vi "Format CSV.vi"(8 "error in (no error)":errorcluster, 9 "delimiter":string=",", 10 "CSV File Input":path, 11 "Original CSV Format":enum16{"Format A", "Format B"}(ring)) -> (0 "error out":errorcluster, 1 "Parcel Length":i32[](array[numeric]), 2 "All Terminal Data":T1(array[cluster]))   [LabVIEW 2017] (continued)
, "42:48.2", "42:48.2", "42:48.3", "42:48.3", "42:48.3", "42:48.4", "42:48.4", "42:48.4", "42:48.5", "42:48.5", "42:48.5", "42:48.6", "42:48.6", "42:48.6", "42:48.7", "42:48.7", "42:48.7", "42:48.8", "42:48.8", "42:48.8", "42:48.9", "42:48.9", "42:48.9", "42:49.0", "42:49.0", "42:49.0", "42:49.1", "42:49.1", "42:49.1", "42:49.2", "42:49.2", "42:49.2", "42:49.3", "42:49.3", "42:49.3", "42:49.4", "42:49.4", "42:49.4", "42:49.5", "42:49.5", "42:49.5", "42:49.6", "42:49.6", "42:49.6", "42:49.7", "42:49.7", "42:49.7", "42:49.8", "42:49.8", "42:49.8", "42:49.9", "42:49.9", "42:49.9", "42:50.0", "42:50.0", "42:50.0", "42:50.1", "42:50.1", "42:50.1", "42:50.2", "42:50.2", "42:50.2", "42:50.3", "42:50.3", "42:50.3", "42:50.4", "42:50.4", "42:50.4", "42:50.5", "42:50.5", "42:50.5", "42:50.6", "42:50.6", "42:50.6", "42:50.7", "42:50.7", "42:50.7", "42:50.8", "42:50.8", "42:50.8", "42:50.9", "42:50.9", "42:50.9", "42:51.0", "42:51.0", "42:51.0", "42:51.1", "42:51.1", "42:51.1", "42:51.2", "42:51.2", "42:51.2", "42:51.3", "42:51.3", "42:51.3", "42:51.4", "42:51.4", "42:51.4", "42:51.5", "42:51.5", "42:51.5", "42:51.6", "42:51.6", "42:51.6", "42:51.7", "42:51.7", "42:51.7", "42:51.8", "42:51.8", "42:51.8", "42:51.9", "42:51.9", "42:51.9", "42:52.0", "42:52.0", "42:52.0", "42:52.1", "42:52.1", "42:52.1", "42:52.2", "42:52.2", "42:52.2", "42:52.3", "42:52.3", "42:52.3", "42:52.4", "42:52.4", "42:52.4", "42:52.5", "42:52.5", "42:52.5", "42:52.6", "42:52.6", "42:52.6", "42:52.7", "42:52.7", "42:52.7", "42:52.8", "42:52.8", "42:52.8", "42:52.9", "42:52.9", "42:52.9", "42:53.0", "42:53.0", "42:53.0", "42:53.1", "42:53.1", "42:53.1", "42:53.2", "42:53.2", "42:53.2", "42:53.3", "42:53.3", "42:53.3", "42:53.4", "42:53.4", "42:53.4", "42:53.5", "42:53.5", "42:53.5", "42:53.6", "42:53.6", "42:53.6", "42:53.7", "42:53.7", "42:53.7", "42:53.8", "42:53.8", "42:53.8", "42:53.9", "42:53.9", "42:53.9", "42:54.0", "42:54.0", "42:54.0", "42:54.1", "42:54.1", "42:54.1", "42:54.2", "42:54.2", "42:54.2", "42:54.3", "42:54.3", "42:54.3", "42:54.4", "42:54.4", "42:54.4", "42:54.5", "42:54.5", "42:54.5", "42:54.6", "42:54.6", "42:54.6", "42:54.7", "42:54.7", "42:54.7", "42:54.8", "42:54.8", "42:54.8", "42:54.9", "42:54.9", "42:54.9", "42:55.0", "42:55.0", "42:55.0", "42:55.1", "42:55.1", "42:55.1", "42:55.2", "42:55.2", "42:55.2", "42:55.3", "42:55.3", "42:55.3", "42:55.4", "42:55.4", "42:55.4", "42:55.5", "42:55.5", "42:55.5", "42:55.6", "42:55.6", "42:55.6", "42:55.7", "42:55.7", "42:55.7", "42:55.8", "42:55.8", "42:55.8", "42:55.9", "42:55.9", "42:55.9", "42:56.0", "42:56.0", "42:56.0", "42:56.1", "42:56.1", "42:56.1", "42:56.2", "42:56.2", "42:56.2", "42:56.3", "42:56.3", "42:56.3", "42:56.4", "42:56.4", "42:56.4", "42:56.5", "42:56.5", "42:56.5", "42:56.6", "42:56.6", "42:56.6", "42:56.7", "42:56.7", "42:56.7", "42:56.8", "42:56.8", "42:56.8", "42:56.9", "42:56.9", "42:56.9", "42:57.0", "42:57.0", "42:57.0", "42:57.1", "42:57.1", "42:57.1", "42:57.2", "42:57.2", "42:57.2", "42:57.3", "42:57.3", "42:57.3", "42:57.4", "42:57.4", "42:57.4", "42:57.5", "42:57.5", "42:57.5", "42:57.6", "42:57.6", "42:57.6", "42:57.7", "42:57.7", "42:57.7", "42:57.8", "42:57.8", "42:57.8", "42:57.9", "42:57.9", "42:57.9", "42:58.0", "42:58.0", "42:58.0", "42:58.1", "42:58.1", "42:58.1", "42:58.2", "42:58.2", "42:58.2", "42:58.3", "42:58.3", "42:58.3", "42:58.4", "42:58.4", "42:58.4", "42:58.5", "42:58.5", "42:58.5", "42:58.6", "42:58.6", "42:58.6", "42:58.7", "42:58.7", "42:58.7", "42:58.8", "42:58.8", "42:58.8", "42:58.9", "42:58.9", "42:58.9", "42:59.0", "42:59.0", "42:59.0", "42:59.1", "42:59.1", "42:59.1", "42:59.2", "42:59.2", "42:59.2", "42:59.3", "42:59.3", "42:59.3", "42:59.4", "42:59.4", "42:59.4", "42:59.5", "42:59.5", "42:59.5", "42:59.6", "42:59.6", "42:59.6", "42:59.7", "42:59.7", "42:59.7", "42:59.8", "42:59.8", "42:59.8", "42:59.9", "42:59.9", "42:59.9", "43:00.0", "43:00.0", "43:00.0", "43:00.1", "43:00.1", "43:00.1", "43:00.2", "43:00.2", "43:00.2", "43:00.3", "43:00.3", "43:00.3", "43:00.4", "43:00.4", "43:00.4", "43:00.5", "43:00.5", "43:00.5", "43:00.6", "43:00.6", "43:00.6", "43:00.7", "43:00.7", "43:00.7", "43:00.8", "43:00.8", "43:00.8", "43:00.9", "43:00.9", "43:00.9", "43:01.0", "43:01.0", "43:01.0", "43:01.1", "43:01.1", "43:01.1", "43:01.2", "43:01.2", "43:01.2", "43:01.3", "43:01.3", "43:01.3", "43:01.4", "43:01.4", "43:01.4", "43:01.5", "43:01.5", "43:01.5", "43:01.6", "43:01.6", "43:01.6", "43:01.7", "43:01.7", "43:01.7", "43:01.8", "43:01.8", "43:01.8", "43:01.9", "43:01.9", "43:01.9", "43:02.0", "43:02.0", "43:02.0", "43:02.1", "43:02.1", "43:02.1", "43:02.2", "43:02.2", "43:02.2", "43:02.3", "43:02.3", "43:02.3", "43:02.4", "43:02.4", "43:02.4", "43:02.5", "43:02.5", "43:02.5", "43:02.6", "43:02.6", "43:02.6", "43:02.7", "43:02.7", "43:02.7", "43:02.8", "43:02.8", "43:02.8", "43:02.9", "43:02.9", "43:02.9", "43:03.0", "43:03.0", "43:03.0", "43:03.1", "43:03.1", "43:03.1", "43:03.2", "43:03.2", "43:03.2", "43:03.3", "43:03.3", "43:03.3", "43:03.4", "43:03.4", "43:03.4", "43:03.5", "43:03.5", "43:03.5", "43:03.6", "43:03.6", "43:03.6", "43:03.7", "43:03.7", "43:03.7", "43:03.8", "43:03.8", "43:03.8", "43:03.9", "43:03.9", "43:03.9", "43:04.0", "43:04.0", "43:04.0", "43:04.1", "43:04.1", "43:04.1", "43:04.2", "43:04.2", "43:04.2", "43:04.3", "43:04.3", "43:04.3", "43:04.4", "43:04.4", "43:04.4", "43:04.5", "43:04.5", "43:04.5", "43:04.6", "43:04.6", "43:04.6", "43:04.7", "43:04.7", "43:04.7", "43:04.8", "43:04.8", "43:04.8", "43:04.9", "43:04.9", "43:04.9", "43:05.0", "43:05.0", "43:05.0", "43:05.1", "43:05.1", "43:05.1", "43:05.2", "43:05.2", "43:05.2", "43:05.3", "43:05.3", "43:05.3", "43:05.4", "43:05.4", "43:05.4", "43:05.5", "43:05.5", "43:05.5", "43:05.6", "43:05.6", "43:05.6", "43:05.7", "43:05.7", "43:05.7", "43:05.8", "43:05.8", "43:05.8", "43:05.9", "43:05.9", "43:05.9", "43:06.0", "43:06.0", "43:06.0", "43:06.1", "43:06.1", "43:06.1", "43:06.2", "43:06.2", "43:06.2", "43:06.3", "43:06.3", "43:06.3", "43:06.4", "43:06.4", "43:06.4", "43:06.5", "43:06.5", "43:06.5", "43:06.6", "43:06.6", "43:06.6", "43:06.7", "43:06.7", "43:06.7", "43:06.8", "43:06.8", "43:06.8", "43:06.9", "43:06.9", "43:06.9", "43:07.0", "43:07.0", "43:07.0", "43:07.1", "43:07.1", "43:07.1", "43:07.2", "43:07.2", "43:07.2", "43:07.3", "43:07.3", "43:07.3", "43:07.4", "43:07.4", "43:07.4", "43:07.5", "43:07.5", "43:07.5", "43:07.6", "43:07.6", "43:07.6", "43:07.7", "43:07.7", "43:07.7", "43:07.8", "43:07.8", "43:07.8", "43:07.9", "43:07.9", "43:07.9", "43:08.0", "43:08.0", "43:08.0", "43:08.1", "43:08.1", "43:08.1", "43:08.2", "43:08.2", "43:08.2", "43:08.3", "43:08.3", "43:08.3", "43:08.4", "43:08.4", "43:08.4", "43:08.5", "43:08.5", "43:08.5", "43:08.6", "43:08.6", "43:08.6", "43:08.7", "43:08.7", "43:08.7", "43:08.8", "43:08.8", "43:08.8", "43:08.9", "43:08.9", "43:08.9", "43:09.0", "43:09.0", "43:09.0", "43:09.1", "43:09.1", "43:09.1", "43:09.2", "43:09.2", "43:09.2", "43:09.3", "43:09.3", "43:09.3", "43:09.4", "43:09.4", "43:09.4", "43:09.5", "43:09.5", "43:09.5", "43:09.6", "43:09.6", "43:09.6", "43:09.7", "43:09.7", "43:09.7", "43:09.8", "43:09.8", "43:09.8", "43:09.9", "43:09.9", "43:09.9", "43:10.0", "43:10.0", "43:10.0", "43:10.1", "43:10.1", "43:10.1", "43:10.2", "43:10.2", "43:10.2", "43:10.3", "43:10.3", "43:10.3", "43:10.4", "43:10.4", "43:10.4", "43:10.5", "43:10.5", "43:10.5", "43:10.6", "43:10.6", "43:10.6", "43:10.7", "43:10.7", "43:10.7", "43:10.8", "43:10.8", "43:10.8", "43:10.9", "43:10.9", "43:10.9", "43:11.0", "43:11.0", "43:11.0", "43:11.1", "43:11.1", "43:11.1", "43:11.2", "43:11.2", "43:11.2", "43:11.3", "43:11.3", "43:11.3", "43:11.4", "43:11.4", "43:11.4", "43:11.5", "43:11.5", "43:11.5", "43:11.6", "43:11.6", "43:11.6", "43:11.7", "43:11.7", "43:11.7", "43:11.8", "43:11.8", "43:11.8", "43:11.9", "43:11.9", "43:11.9", "43:12.0", "43:12.0", "43:12.0", "43:12.1", "43:12.1", "43:12.1", "43:12.2", "43:12.2", "43:12.2", "43:12.3", "43:12.3", "43:12.3", "43:12.4", "43:12.4", "43:12.4", "43:12.5", "43:12.5", "43:12.5", "43:12.6", "43:12.6", "43:12.6", "43:12.7", "43:12.7", "43:12.7", "43:12.8", "43:12.8", "43:12.8", "43:12.9", "43:12.9", "43:12.9", "43:13.0", "43:13.0", "43:13.0", "43:13.1", "43:13.1", "43:13.1", "43:13.2", "43:13.2", "43:13.2", "43:13.3", "43:13.3", "43:13.3", "43:13.4", "43:13.4", "43:13.4", "43:13.5", "43:13.5", "43:13.5", "43:13.6", "43:13.6", "43:13.6", "43:13.7", "43:13.7", "43:13.7", "43:13.8", "43:13.8", "43:13.8", "43:13.9", "43:13.9", "43:13.9", "43:14.0", "43:14.0", "43:14.0", "43:14.1", "43:14.1", "43:14.1", "43:14.2", "43:14.2", "43:14.2", "43:14.3", "43:14.3", "43:14.3", "43:14.4", "43:14.4", "43:14.4", "43:14.5", "43:14.5", "43:14.5", "43:14.6", "43:14.6", "43:14.6", "43:14.7", "43:14.7", "43:14.7", "43:14.8", "43:14.8", "43:14.8", "43:14.9", "43:14.9", "43:14.9", "43:15.0", "43:15.0", "43:15.0", "43:15.1", "43:15.1", "43:15.1", "43:15.2", "43:15.2", "43:15.2", "43:15.3", "43:15.3", "43:15.3", "43:15.4", "43:15.4", "43:15.4", "43:15.5", "43:15.5", "43:15.5", "43:15.6", "43:15.6", "43:15.6", "43:15.7", "43:15.7", "43:15.7", "43:15.8", "43:15.8", "43:15.8", "43:15.9", "43:15.9", "43:15.9", "43:16.0", "43:16.0", "43:16.0", "43:16.1", "43:16.1", "43:16.1", "43:16.2", "43:16.2", "43:16.2", "43:16.3", "43:16.3", "43:16.3", "43:16.4", "43:16.4", "43:16.4", "43:16.5", "43:16.5", "43:16.5", "43:16.6", "43:16.6", "43:16.6", "43:16.7", "43:16.7", "43:16.7", "43:16.8", "43:16.8", "43:16.8", "43:16.9", "43:16.9", "43:16.9", "43:17.0", "43:17.0", "43:17.0", "43:17.1", "43:17.1", "43:17.1", "43:17.2", "43:17.2", "43:17.2", "43:17.3", "43:17.3", "43:17.3", "43:17.4", "43:17.4", "43:17.4", "43:17.5", "43:17.5", "43:17.5", "43:17.6", "43:17.6", "43:17.6", "43:17.7", "43:17.7", "43:17.7", "43:17.8", "43:17.8", "43:17.8", "43:17.9", "43:17.9", "43:17.9", "43:18.0", "43:18.0", "43:18.0", "43:18.1", "43:18.1", "43:18.1", "43:18.2", "43:18.2", "43:18.2", "43:18.3", "43:18.3", "43:18.3", "43:18.4", "43:18.4", "43:18.4", "43:18.5", "43:18.5", "43:18.5", "43:18.6", "43:18.6", "43:18.6", "43:18.7", "43:18.7", "43:18.7", "43:18.8", "43:18.8", "43:18.8", "43:18.9", "43:18.9", "43:18.9", "43:19.0", "43:19.0", "43:19.0", "43:19.1", "43:19.1", "43:19.1", "43:19.2", "43:19.2", "43:19.2", "43:19.3", "43:19.3", "43:19.3", "43:19.4", "43:19.4", "43:19.4", "43:19.5", "43:19.5", "43:19.5", "43:19.6", "43:19.6", "43:19.6", "43:19.7", "43:19.7", "43:19.7", "43:19.8", "43:19.8", "43:19.8", "43:19.9", "43:19.9", "43:19.9", "43:20.0", "43:20.0", "43:20.0", "43:20.1", "43:20.1", "43:20.1", "43:20.2", "43:20.2", "43:20.2", "43:20.3", "43:20.3", "43:20.3", "43:20.4", "43:20.4", "43:20.4", "43:20.5", "43:20.5", "43:20.5", "43:20.6", "43:20.6", "43:20.6", "43:20.7", "43:20.7", "43:20.7", "43:20.8", "43:20.8", "43:20.8", "43:20.9", "43:20.9", "43:20.9", "43:21.0", "43:21.0", "43:21.0", "43:21.1", "43:21.1", "43:21.1", "43:21.2", "43:21.2", "43:21.2", "43:21.3", "43:21.3", "43:21.3", "43:21.4", "43:21.4", "43:21.4", "43:21.5", "43:21.5", "43:21.5", "43:21.6", "43:21.6", "43:21.6", "43:21.7", "43:21.7", "43:21.7", "43:21.8", "43:21.8", "43:21.8", "43:21.9", "43:21.9", "43:21.9", "43:22.0", "43:22.0", "43:22.0", "43:22.1", "43:22.1", "43:22.1", "43:22.2", "43:22.2", "43:22.2", "43:22.3", "43:22.3", "43:22.3", "43:22.4", "43:22.4", "43:22.4", "43:22.5", "43:22.5", "43:22.5", "43:22.6", "43:22.6", "43:22.6", "43:22.7", "43:22.7", "43:22.7", "43:22.8", "43:22.8", "43:22.8", "43:22.9", "43:22.9", "43:22.9", "43:23.0", "43:23.0", "43:23.0", "43:23.1", "43:23.1", "43:23.1", "43:23.2", "43:23.2", "43:23.2", "43:23.3", "43:23.3", "43:23.3", "43:23.4", "43:23.4", "43:23.4", "43:23.5", "43:23.5", "43:23.5", "43:23.6", "43:23.6", "43:23.6", "43:23.7", "43:23.7", "43:23.7", "43:23.8", "43:23.8", "43:23.8", "43:23.9", "43:23.9", "43:23.9", "43:24.0", "43:24.0", "43:24.0", "43:24.1", "43:24.1", "43:24.1", "43:24.2", "43:24.2", "43:24.2", "43:24.3", "43:24.3", "43:24.3", "43:24.4", "43:24.4", "43:24.4", "43:24.5", "43:24.5", "43:24.5", "43:24.6", "43:24.6", "43:24.6", "43:24.7", "43:24.7", "43:24.7", "43:24.8", "43:24.8", "43:24.8", "43:24.9", "43:24.9", "43:24.9", "43:25.0", "43:25.0", "43:25.0", "43:25.1", "43:25.1", "43:25.1", "43:25.2", "43:25.2", "43:25.2", "43:25.3", "43:25.3", "43:25.3", "43:25.4", "43:25.4", "43:25.4", "43:25.5", "43:25.5", "43:25.5", "43:25.6", "43:25.6", "43:25.6", "43:25.7", "43:25.7", "43:25.7", "43:25.8", "43:25.8", "43:25.8", "43:25.9", "43:25.9", "43:25.9", "43:26.0", "43:26.0", "43:26.0", "43:26.1", "43:26.1", "43:26.1", "43:26.2", "43:26.2", "43:26.2", "43:26.3", "43:26.3", "43:26.3", "43:26.4", "43:26.4", "43:26.4", "43:26.5", "43:26.5", "43:26.5", "43:26.6", "43:26.6", "43:26.6", "43:26.7", "43:26.7", "43:26.7", "43:26.8", "43:26.8", "43:26.8", "43:26.9", "43:26.9", "43:26.9", "43:27.0", "43:27.0", "43:27.0", "43:27.1", "43:27.1", "43:27.1", "43:27.2", "43:27.2", "43:27.2", "43:27.3", "43:27.3", "43:27.3", "43:27.4", "43:27.4", "43:27.4", "43:27.5", "43:27.5", "43:27.5", "43:27.6", "43:27.6", "43:27.6", "43:27.7", "43:27.7", "43:27.7", "43:27.8", "43:27.8", "43:27.8", "43:27.9", "43:27.9", "43:27.9", "43:28.0", "43:28.0", "43:28.0", "43:28.1", "43:28.1", "43:28.1", "43:28.2", "43:28.2", "43:28.2", "43:28.3", "43:28.3", "43:28.3", "43:28.4", "43:28.4", "43:28.4", "43:28.5", "43:28.5", "43:28.5", "43:28.6", "43:28.6", "43:28.6", "43:28.7", "43:28.7", "43:28.7", "43:28.8", "43:28.8", "43:28.8", "43:28.9", "43:28.9", "43:28.9", "43:29.0", "43:29.0", "43:29.0", "43:29.1", "43:29.1", "43:29.1", "43:29.2", "43:29.2", "43:29.2", "43:29.3", "43:29.3", "43:29.3", "43:29.4", "43:29.4", "43:29.4", "43:29.5", "43:29.5", "43:29.5", "43:29.6", "43:29.6", "43:29.6", "43:29.7", "43:29.7", "43:29.7", "43:29.8", "43:29.8", "43:29.8", "43:29.9", "43:29.9", "43:29.9", "43:30.0", "43:30.0", "43:30.0", "43:30.1", "43:30.1", "43:30.1", "43:30.2", "43:30.2", "43:30.2", "43:30.3", "43:30.3", "43:30.3", "43:30.4", "43:30.4", "43:30.4", "43:30.5", "43:30.5", "43:30.5", "43:30.6", "43:30.6", "43:30.6", "43:30.7", "43:30.7", "43:30.7", "43:30.8", "43:30.8", "43:30.8", "43:30.9", "43:30.9", "43:30.9", "43:31.0", "43:31.0", "43:31.0", "43:31.1", "43:31.1", "43:31.1", "43:31.2", "43:31.2", "43:31.2", "43:31.3", "43:31.3", "43:31.3", "43:31.4", "43:31.4", "43:31.4", "43:31.5", "43:31.5", "43:31.5", "43:31.6", "43:31.6", "43:31.6", "43:31.7", "43:31.7", "43:31.7", "43:31.8", "43:31.8", "43:31.8", "43:31.9", "43:31.9", "43:31.9", "43:32.0", "43:32.0", "43:32.0", "43:32.1", "43:32.1", "43:32.1", "43:32.2", "43:32.2", "43:32.2", "43:32.3", "43:32.3", "43:32.3", "43:32.4", "43:32.4", "43:32.4", "43:32.5", "43:32.5", "43:32.5", "43:32.6", "43:32.6", "43:32.6", "43:32.7", "43:32.7", "43:32.7", "43:32.8", "43:32.8", "43:32.8", "43:32.9", "43:32.9", "43:32.9", "43:33.0", "43:33.0", "43:33.0", "43:33.1", "43:33.1", "43:33.1", "43:33.2", "43:33.2", "43:33.2", "43:33.3", "43:33.3", "43:33.3", "43:33.4", "43:33.4", "43:33.4", "43:33.5", "43:33.5", "43:33.5", "43:33.6", "43:33.6", "43:33.6", "43:33.7", "43:33.7", "43:33.7", "43:33.8", "43:33.8", "43:33.8", "43:33.9", "43:33.9", "43:33.9", "43:34.0", "43:34.0", "43:34.0", "43:34.1", "43:34.1", "43:34.1", "43:34.2", "43:34.2", "43:34.2", "43:34.3", "43:34.3", "43:34.3", "43:34.4", "43:34.4", "43:34.4", "43:34.5", "43:34.5", "43:34.5", "43:34.6", "43:34.6", "43:34.6", "43:34.7", "43:34.7", "43:34.7", "43:34.8", "43:34.8", "43:34.8", "43:34.9", "43:34.9", "43:34.9", "43:35.0", "43:35.0", "43:35.0", "43:35.1", "43:35.1", "43:35.1", "43:35.2", "43:35.2", "43:35.2", "43:35.3", "43:35.3", "43:35.3", "43:35.4", "43:35.4", "43:35.4", "43:35.5", "43:35.5", "43:35.5", "43:35.6", "43:35.6", "43:35.6", "43:35.7", "43:35.7", "43:35.7", "43:35.8", "43:35.8", "43:35.8", "43:35.9", "43:35.9", "43:35.9", "43:36.0", "43:36.0", "43:36.0", "43:36.1", "43:36.1", "43:36.1", "43:36.2", "43:36.2", "43:36.2", "43:36.3", "43:36.3", "43:36.3", "43:36.4", "43:36.4", "43:36.4", "43:36.5", "43:36.5", "43:36.5", "43:36.6", "43:36.6", "43:36.6", "43:36.7", "43:36.7", "43:36.7", "43:36.8", "43:36.8", "43:36.8", "43:36.9", "43:36.9", "43:36.9", "43:37.0", "43:37.0", "43:37.0", "43:37.1", "43:37.1", "43:37.1", "43:37.2", "43:37.2", "43:37.2", "43:37.3", "43:37.3", "43:37.3", "43:37.4", "43:37.4", "43:37.4", "43:37.5", "43:37.5", "43:37.5", "43:37.6", "43:37.6", "43:37.6", "43:37.7", "43:37.7", "43:37.7", "43:37.8", "43:37.8", "43:37.8", "43:37.9", "43:37.9", "43:37.9", "43:38.0", "43:38.0", "43:38.0", "43:38.1", "43:38.1", "43:38.1", "43:38.2", "43:38.2", "43:38.2", "43:38.3", "43:38.3", "43:38.3", "43:38.4", "43:38.4", "43:38.4", "43:38.5", "43:38.5", "43:38.5", "43:38.6", "43:38.6", "43:38.6", "43:38.7", "43:38.7", "43:38.7", "43:38.8", "43:38.8", "43:38.8", "43:38.9", "43:38.9", "43:38.9", "43:39.0", "43:39.0", "43:39.0", "43:39.1", "43:39.1", "43:39.1", "43:39.2", "43:39.2", "43:39.2", "43:39.3", "43:39.3", "43:39.3", "43:39.4", "43:39.4", "43:39.4", "43:39.5", "43:39.5", "43:39.5", "43:39.6", "43:39.6", "43:39.6", "43:39.7", "43:39.7", "43:39.7", "43:39.8", "43:39.8", "43:39.8", "43:39.9", "43:39.9", "43:39.9", "43:40.0", "43:40.0", "43:40.0", "43:40.1", "43:40.1", "43:40.1", "43:40.2", "43:40.2", "43:40.2", "43:40.3", "43:40.3", "43:40.3", "43:40.4", "43:40.4", "43:40.4", "43:40.5", "43:40.5", "43:40.5", "43:40.6", "43:40.6", "43:40.6", "43:40.7", "43:40.7", "43:40.7", "43:40.8", "43:40.8", "43:40.8", "43:40.9", "43:40.9", "43:40.9", "43:41.0", "43:41.0", "43:41.0", "43:41.1", "43:41.1", "43:41.1", "43:41.2", "43:41.2", "43:41.2", "43:41.3", "43:41.3", "43:41.3", "43:41.4", "43:41.4", "43:41.4", "43:41.5", "43:41.5", "43:41.5", "43:41.6", "43:41.6", "43:41.6", "43:41.7", "43:41.7", "43:41.7", "43:41.8", "43:41.8", "43:41.8", "43:41.9", "43:41.9", "43:41.9", "43:42.0", "43:42.0", "43:42.0", "43:42.1", "43:42.1", "43:42.1", "43:42.2", "43:42.2", "43:42.2", "43:42.3", "43:42.3", "43:42.3", "43:42.4", "43:42.4", "43:42.4", "43:42.5", "43:42.5", "43:42.5", "43:42.6", "43:42.6", "43:42.6", "43:42.7", "43:42.7", "43:42.7", "43:42.8", "43:42.8", "43:42.8", "43:42.9", "43:42.9", "43:42.9", "43:43.0", "43:43.0", "43:43.0", "43:43.1", "43:43.1", "43:43.1", "43:43.2", "43:43.2", "43:43.2", "43:43.3", "43:43.3", "43:43.3", "43:43.4", "43:43.4", "43:43.4", "43:43.5", "43:43.5", "43:43.5", "43:43.6", "43:43.6", "43:43.6", "43:43.7", "43:43.7", "43:43.7", "43:43.8", "43:43.8", "43:43.8", "43:43.9", "43:43.9", "43:43.9", "43:44.0", "43:44.0", "43:44.0", "43:44.1", "43:44.1", "43:44.1", "43:44.2", "43:44.2", "43:44.2", "43:44.3", "43:44.3", "43:44.3", "43:44.4", "43:44.4", "43:44.4", "43:44.5", "43:44.5", "43:44.5", "43:44.6", "43:44.6", "43:44.6", "43:44.7", "43:44.7", "43:44.7", "43:44.8", "43:44.8", "43:44.8", "43:44.9", "43:44.9", "43:44.9", "43:45.0", "43:45.0", "43:45.0", "43:45.1", "43:45.1", "43:45.1", "43:45.2", "43:45.2", "43:45.2", "43:45.3", "43:45.3", "43:45.3", "43:45.4", "43:45.4", "43:45.4", "43:45.5", "43:45.5", "43:45.5", "43:45.6", "43:45.6", "43:45.6", "43:45.7", "43:45.7", "43:45.7", "43:45.8", "43:45.8", "43:45.8", "43:45.9", "43:45.9", "43:45.9", "43:46.0", "43:46.0", "43:46.0", "43:46.1", "43:46.1", "43:46.1", "43:46.2", "43:46.2", "43:46.2", "43:46.3", "43:46.3", "43:46.3", "43:46.4", "43:46.4", "43:46.4", "43:46.5", "43:46.5", "43:46.5", "43:46.6", "43:46.6", "43:46.6", "43:46.7", "43:46.7", "43:46.7", "43:46.8", "43:46.8", "43:46.8", "43:46.9", "43:46.9", "43:46.9", "43:47.0", "43:47.0", "43:47.0", "43:47.1", "43:47.1", "43:47.1", "43:47.2", "43:47.2", "43:47.2", "43:47.3", "43:47.3", "43:47.3", "43:47.4", "43:47.4", "43:47.4", "43:47.5", "43:47.5", "43:47.5", "43:47.6", "43:47.6", "43:47.6", "43:47.7", "43:47.7", "43:47.7", "43:47.8", "43:47.8", "43:47.8", "43:47.9", "43:47.9", "43:47.9", "43:48.0", "43:48.0", "43:48.0", "43:48.1", "43:48.1", "43:48.1", "43:48.2", "43:48.2", "43:48.2", "43:48.3", "43:48.3", "43:48.3", "43:48.4", "43:48.4", "43:48.4", "43:48.5", "43:48.5", "43:48.5", "43:48.6", "43:48.6", "43:48.6", "43:48.7", "43:48.7", "43:48.7", "43:48.8", "43:48.8", "43:48.8", "43:48.9", "43:48.9", "43:48.9", "43:49.0", "43:49.0", "43:49.0", "43:49.1", "43:49.1", "43:49.1", "43:49.2", "43:49.2", "43:49.2", "43:49.3", "43:49.3", "43:49.3", "43:49.4", "43:49.4", "43:49.4", "43:49.5", "43:49.5", "43:49.5", "43:49.6", "43:49.6", "43:49.6", "43:49.7", "43:49.7", "43:49.7", "43:49.8", "43:49.8", "43:49.8", "43:49.9", "43:49.9", "43:49.9", "43:50.0", "43:50.0", "43:50.0", "43:50.1", "43:50.1", "43:50.1", "43:50.2", "43:50.2", "43:50.2", "43:50.3", "43:50.3", "43:50.3", "43:50.4", "43:50.4", "43:50.4", "43:50.5", "43:50.5", "43:50.5", "43:50.6", "43:50.6", "43:50.6", "43:50.7", "43:50.7", "43:50.7", "43:50.8", "43:50.8", "43:50.8", "43:50.9", "43:50.9", "43:50.9", "43:51.0", "43:51.0", "43:51.0", "43:51.1", "43:51.1", "43:51.1", "43:51.2", "43:51.2", "43:51.2", "43:51.3", "43:51.3", "43:51.3", "43:51.4", "43:51.4", "43:51.4", "43:51.5", "43:51.5", "43:51.5", "43:51.6", "43:51.6", "43:51.6", "43:51.7", "43:51.7", "43:51.7", "43:51.8", "43:51.8", "43:51.8", "43:51.9", "43:51.9", "43:51.9", "43:52.0", "43:52.0", "43:52.0", "43:52.1", "43:52.1", "43:52.1", "43:52.2", "43:52.2", "43:52.2", "43:52.3", "43:52.3", "43:52.3", "43:52.4", "43:52.4", "43:52.4", "43:52.5", "43:52.5", "43:52.5", "43:52.6", "43:52.6", "43:52.6", "43:52.7", "43:52.7", "43:52.7", "43:52.8", "43:52.8", "43:52.8", "43:52.9", "43:52.9", "43:52.9", "43:53.0", "43:53.0", "43:53.0", "43:53.1", "43:53.1", "43:53.1", "43:53.2", "43:53.2", "43:53.2", "43:53.3", "43:53.3", "43:53.3", "43:53.4", "43:53.4", "43:53.4", "43:53.5", "43:53.5", "43:53.5", "43:53.6", "43:53.6", "43:53.6", "43:53.7", "43:53.7", "43:53.7", "43:53.8", "43:53.8", "43:53.8", "43:53.9", "43:53.9", "43:53.9", "43:54.0", "43:54.0", "43:54.0", "43:54.1", "43:54.1", "43:54.1", "43:54.2", "43:54.2", "43:54.2", "43:54.3", "43:54.3", "43:54.3", "43:54.4", "43:54.4", "43:54.4", "43:54.5", "43:54.5", "43:54.5", "43:54.6", "43:54.6", "43:54.6", "43:54.7", "43:54.7", "43:54.7", "43:54.8", "43:54.8", "43:54.8", "43:54.9", "43:54.9", "43:54.9", "43:55.0", "43:55.0", "43:55.0", "43:55.1", "43:55.1", "43:55.1", "43:55.2", "43:55.2", "43:55.2", "43:55.3", "43:55.3", "43:55.3", "43:55.4", "43:55.4", "43:55.4", "43:55.5", "43:55.5", "43:55.5", "43:55.6", "43:55.6", "43:55.6", "43:55.7", "43:55.7", "43:55.7", "43:55.8", "43:55.8", "43:55.8", "43:55.9", "43:55.9", "43:55.9", "43:56.0", "43:56.0", "43:56.0", "43:56.1", "43:56.1", "43:56.1", "43:56.2", "43:56.2", "43:56.2", "43:56.3", "43:56.3", "43:56.3", "43:56.4", "43:56.4", "43:56.4", "43:56.5", "43:56.5", "43:56.5", "43:56.6", "43:56.6", "43:56.6", "43:56.7", "43:56.7", "43:56.7", "43:56.8", "43:56.8", "43:56.8", "43:56.9", "43:56.9", "43:56.9", "43:57.0", "43:57.0", "43:57.0", "43:57.1", "43:57.1", "43:57.1", "43:57.2", "43:57.2", "43:57.2", "43:57.3", "43:57.3", "43:57.3", "43:57.4", "43:57.4", "43:57.4", "43:57.5", "43:57.5", "43:57.5", "43:57.6", "43:57.6", "43:57.6", "43:57.7", "43:57.7", "43:57.7", "43:57.8", "43:57.8", "43:57.8", "43:57.9", "43:57.9", "43:57.9", "43:58.0", "43:58.0", "43:58.0", "43:58.1", "43:58.1", "43:58.1", "43:58.2", "43:58.2", "43:58.2", "43:58.3", "43:58.3", "43:58.3", "43:58.4", "43:58.4", "43:58.4", "43:58.5", "43:58.5", "43:58.5", "43:58.6", "43:58.6", "43:58.6", "43:58.7", "43:58.7", "43:58.7", "43:58.8", "43:58.8", "43:58.8", "43:58.9", "43:58.9", "43:58.9", "43:59.0", "43:59.0", "43:59.0", "43:59.1", "43:59.1", "43:59.1", "43:59.2", "43:59.2", "43:59.2", "43:59.3", "43:59.3", "43:59.3", "43:59.4", "43:59.4", "43:59.4", "43:59.5", "43:59.5", "43:59.5", "43:59.6", "43:59.6", "43:59.6", "43:59.7", "43:59.7", "43:59.7", "43:59.8", "43:59.8", "43:59.8", "43:59.9", "43:59.9", "43:59.9", "44:00.0", "44:00.0", "44:00.0", "44:00.1", "44:00.1", "44:00.1", "44:00.2", "44:00.2", "44:00.2", "44:00.3", "44:00.3", "44:00.3", "44:00.4", "44:00.4", "44:00.4", "44:00.5", "44:00.5", "44:00.5", "44:00.6", "44:00.6", "44:00.6", "44:00.7", "44:00.7", "44:00.7", "44:00.8", "44:00.8", "44:00.8", "44:00.9", "44:00.9", "44:00.9", "44:01.0", "44:01.0", "44:01.0", "44:01.1", "44:01.1", "44:01.1", "44:01.2", "44:01.2", "44:01.2", "44:01.3", "44:01.3", "44:01.3", "44:01.4", "44:01.4", "44:01.4", "44:01.5", "44:01.5", "44:01.5", "44:01.6", "44:01.6", "44:01.6", "44:01.7", "44:01.7", "44:01.7", "44:01.8", "44:01.8", "44:01.8", "44:01.9", "44:01.9", "44:01.9", "44:02.0", "44:02.0", "44:02.0", "44:02.1", "44:02.1", "44:02.1", "44:02.2", "44:02.2", "44:02.2", "44:02.3", "44:02.3", "44:02.3", "44:02.4", "44:02.4", "44:02.4", "44:02.5", "44:02.5", "44:02.5", "44:02.6", "44:02.6", "44:02.6", "44:02.7", "44:02.7", "44:02.7", "44:02.8", "44:02.8", "44:02.8", "44:02.9", "44:02.9", "44:02.9", "44:03.0", "44:03.0", "44:03.0", "44:03.1", "44:03.1", "44:03.1", "44:03.2", "44:03.2", "44:03.2", "44:03.3", "44:03.3", "44:03.3", "44:03.4", "44:03.4", "44:03.4", "44:03.5", "44:03.5", "44:03.5", "44:03.6", "44:03.6", "44:03.6", "44:03.7", "44:03.7", "44:03.7", "44:03.8", "44:03.8", "44:03.8", "44:03.9", "44:03.9", "44:03.9", "44:04.0", "44:04.0", "44:04.0", "44:04.1", "44:04.1", "44:04.1", "44:04.2", "44:04.2", "44:04.2", "44:04.3", "44:04.3", "44:04.3", "44:04.4", "44:04.4", "44:04.4", "44:04.5", "44:04.5", "44:04.5", "44:04.6", "44:04.6", "44:04.6", "44:04.7", "44:04.7", "44:04.7", "44:04.8", "44:04.8", "44:04.8", "44:04.9", "44:04.9", "44:04.9", "44:05.0", "44:05.0", "44:05.0", "44:05.1", "44:05.1", "44:05.1", "44:05.2", "44:05.2", "44:05.2", "44:05.3", "44:05.3", "44:05.3", "44:05.4", "44:05.4", "44:05.4", "44:05.5", "44:05.5", "44:05.5", "44:05.6", "44:05.6", "44:05.6", "44:05.7", "44:05.7", "44:05.7", "44:05.8", "44:05.8", "44:05.8", "44:05.9", "44:05.9", "44:05.9", "44:06.0", "44:06.0", "44:06.0", "44:06.1", "44:06.1", "44:06.1", "44:06.2", "44:06.2", "44:06.2", "44:06.3", "44:06.3", "44:06.3", "44:06.4", "44:06.4", "44:06.4", "44:06.5", "44:06.5", "44:06.5", "44:06.6", "44:06.6", "44:06.6", "44:06.7", "44:06.7", "44:06.7", "44:06.8", "44:06.8", "44:06.8", "44:06.9", "44:06.9", "44:06.9", "44:07.0", "44:07.0", "44:07.0", "44:07.1", "44:07.1", "44:07.1", "44:07.2", "44:07.2", "44:07.2", "44:07.3", "44:07.3", "44:07.3", "44:07.4", "44:07.4", "44:07.4", "44:07.5", "44:07.5", "44:07.5", "44:07.6", "44:07.6", "44:07.6", "44:07.7", "44:07.7", "44:07.7", "44:07.8", "44:07.8", "44:07.8", "44:07.9", "44:07.9", "44:07.9", "44:08.0", "44:08.0", "44:08.0", "44:08.1", "44:08.1", "44:08.1", "44:08.2", "44:08.2", "44:08.2", "44:08.3", "44:08.3", "44:08.3", "44:08.4", "44:08.4", "44:08.4", "44:08.5", "44:08.5", "44:08.5", "44:08.6", "44:08.6", "44:08.6", "44:08.7", "44:08.7", "44:08.7", "44:08.8", "44:08.8", "44:08.8", "44:08.9", "44:08.9", "44:08.9", "44:09.0", "44:09.0", "44:09.0", "44:09.1", "44:09.1", "44:09.1", "44:09.2", "44:09.2", "44:09.2", "44:09.3", "44:09.3", "44:09.3", "44:09.4", "44:09.4", "44:09.4", "44:09.5", "44:09.5", "44:09.5", "44:09.6", "44:09.6", "44:09.6", "44:09.7", "44:09.7", "44:09.7", "44:09.8", "44:09.8", "44:09.8", "44:09.9", "44:09.9", "44:09.9", "44:10.0", "44:10.0", "44:10.0", "44:10.1", "44:10.1", "44:10.1", "44:10.2", "44:10.2", "44:10.2", "44:10.3", "44:10.3", "44:10.3", "44:10.4", "44:10.4", "44:10.4", "44:10.5", "44:10.5", "44:10.5", "44:10.6", "44:10.6", "44:10.6", "44:10.7", "44:10.7", "44:10.7", "44:10.8", "44:10.8", "44:10.8", "44:10.9", "44:10.9", "44:10.9", "44:11.0", "44:11.0", "44:11.0", "44:11.1", "44:11.1", "44:11.1", "44:11.2", "44:11.2", "44:11.2", "44:11.3", "44:11.3", "44:11.3", "44:11.4", "44:11.4", "44:11.4", "44:11.5", "44:11.5", "44:11.5", "44:11.6", "44:11.6", "44:11.6", "44:11.7", "44:11.7", "44:11.7", "44:11.8", "44:11.8", "44:11.8", "44:11.9", "44:11.9", "44:11.9", "44:12.0", "44:12.0", "44:12.0", "44:12.1", "44:12.1", "44:12.1", "44:12.2", "44:12.2", "44:12.2", "44:12.3", "44:12.3", "44:12.3", "44:12.4", "44:12.4", "44:12.4", "44:12.5", "44:12.5", "44:12.5", "44:12.6", "44:12.6", "44:12.6", "44:12.7", "44:12.7", "44:12.7", "44:12.8", "44:12.8", "44:12.8", "44:12.9", "44:12.9", "44:12.9", "44:13.0", "44:13.0", "44:13.0", "44:13.1", "44:13.1", "44:13.1", "44:13.2", "44:13.2", "44:13.2", "44:13.3", "44:13.3", "44:13.3", "44:13.4", "44:13.4", "44:13.4", "44:13.5", "44:13.5", "44:13.5", "44:13.6", "44:13.6", "44:13.6", "44:13.7", "44:13.7", "44:13.7", "44:13.8", "44:13.8", "44:13.8", "44:13.9", "44:13.9", "44:13.9", "44:14.0", "44:14.0", "44:14.0", "44:14.1", "44:14.1", "44:14.1", "44:14.2", "44:14.2", "44:14.2", "44:14.3", "44:14.3", "44:14.3", "44:14.4", "44:14.4", "44:14.4", "44:14.5", "44:14.5", "44:14.5", "44:14.6", "44:14.6", "44:14.6", "44:14.7", "44:14.7", "44:14.7", "44:14.8", "44:14.8", "44:14.8", "44:14.9", "44:14.9", "44:14.9", "44:15.0", "44:15.0", "44:15.0", "44:15.1", "44:15.1", "44:15.1", "44:15.2", "44:15.2", "44:15.2", "44:15.3", "44:15.3", "44:15.3", "44:15.4", "44:15.4", "44:15.4", "44:15.5", "44:15.5", "44:15.5", "44:15.6", "44:15.6", "44:15.6", "44:15.7", "44:15.7", "44:15.7", "44:15.8", "44:15.8", "44:15.8", "44:15.9", "44:15.9", "44:15.9", "44:16.0", "44:16.0", "44:16.0", "44:16.1", "44:16.1", "44:16.1", "44:16.2", "44:16.2", "44:16.2", "44:16.3", "44:16.3", "44:16.3", "44:16.4", "44:16.4", "44:16.4", "44:16.5", "44:16.5", "44:16.5", "44:16.6", "44:16.6", "44:16.6", "44:16.7", "44:16.7", "44:16.7", "44:16.8", "44:16.8", "44:16.8", "44:16.9", "44:16.9", "44:16.9", "44:17.0", "44:17.0", "44:17.0", "44:17.1", "44:17.1", "44:17.1", "44:17.2", "44:17.2", "44:17.2", "44:17.3", "44:17.3", "44:17.3", "44:17.4", "44:17.4", "44:17.4", "44:17.5", "44:17.5", "44:17.5", "44:17.6", "44:17.6", "44:17.6", "44:17.7", "44:17.7", "44:17.7", "44:17.8", "44:17.8", "44:17.8", "44:17.9", "44:17.9", "44:17.9", "44:18.0", "44:18.0", "44:18.0", "44:18.1", "44:18.1", "44:18.1", "44:18.2", "44:18.2", "44:18.2", "44:18.3", "44:18.3", "44:18.3", "44:18.4", "44:18.4", "44:18.4", "44:18.5", "44:18.5", "44:18.5", "44:18.6", "44:18.6", "44:18.6", "44:18.7", "44:18.7", "44:18.7", "44:18.8", "44:18.8", "44:18.8", "44:18.9", "44:18.9", "44:18.9", "44:19.0", "44:19.0", "44:19.0", "44:19.1", "44:19.1", "44:19.1", "44:19.2", "44:19.2", "44:19.2", "44:19.3", "44:19.3", "44:19.3", "44:19.4", "44:19.4", "44:19.4", "44:19.5", "44:19.5", "44:19.5", "44:19.6", "44:19.6", "44:19.6", "44:19.7", "44:19.7", "44:19.7", "44:19.8", "44:19.8", "44:19.8", "44:19.9", "44:19.9", "44:19.9", "44:20.0", "44:20.0", "44:20.0", "44:20.1", "44:20.1", "44:20.1", "44:20.2", "44:20.2", "44:20.2", "44:20.3", "44:20.3", "44:20.3", "44:20.4", "44:20.4", "44:20.4", "44:20.5", "44:20.5", "44:20.5", "44:20.6", "44:20.6", "44:20.6", "44:20.7", "44:20.7", "44:20.7", "44:20.8", "44:20.8", "44:20.8", "44:20.9", "44:20.9", "44:20.9", "44:21.0", "44:21.0", "44:21.0", "44:21.1", "44:21.1", "44:21.1", "44:21.2", "44:21.2", "44:21.2", "44:21.3", "44:21.3", "44:21.3", "44:21.4", "44:21.4", "44:21.4", "44:21.5", "44:21.5", "44:21.5", "44:21.6", "44:21.6", "44:21.6", "44:21.7", "44:21.7", "44:21.7", "44:21.8", "44:21.8", "44:21.8", "44:21.9", "44:21.9", "44:21.9", "44:22.0", "44:22.0", "44:22.0", "44:22.1", "44:22.1", "44:22.1", "44:22.2", "44:22.2", "44:22.2", "44:22.3", "44:22.3", "44:22.3", "44:22.4", "44:22.4", "44:22.4", "44:22.5", "44:22.5", "44:22.5", "44:22.6", "44:22.6", "44:22.6", "44:22.7", "44:22.7", "44:22.7", "44:22.8", "44:22.8", "44:22.8", "44:22.9", "44:22.9", "44:22.9", "44:23.0", "44:23.0", "44:23.0", "44:23.1", "44:23.1", "44:23.1", "44:23.2", "44:23.2", "44:23.2", "44:23.3", "44:23.3", "44:23.3", "44:23.4", "44:23.4", "44:23.4", "44:23.5", "44:23.5", "44:23.5", "44:23.6", "44:23.6", "44:23.6", "44:23.7", "44:23.7", "44:23.7", "44:23.8", "44:23.8", "44:23.8", "44:23.9", "44:23.9", "44:23.9", "44:24.0", "44:24.0", "44:24.0", "44:24.1", "44:24.1", "44:24.1", "44:24.2", "44:24.2", "44:24.2", "44:24.3", "44:24.3", "44:24.3", "44:24.4", "44:24.4", "44:24.4", "44:24.5", "44:24.5", "44:24.5", "44:24.6", "44:24.6", "44:24.6", "44:24.7", "44:24.7", "44:24.7", "44:24.8", "44:24.8", "44:24.8", "44:24.9", "44:24.9", "44:24.9", "44:25.0", "44:25.0", "44:25.0", "44:25.1", "44:25.1", "44:25.1", "44:25.2", "44:25.2", "44:25.2", "44:25.3", "44:25.3", "44:25.3", "44:25.4", "44:25.4", "44:25.4", "44:25.5", "44:25.5", "44:25.5", "44:25.6", "44:25.6", "44:25.6", "44:25.7", "44:25.7", "44:25.7", "44:25.8", "44:25.8", "44:25.8", "44:25.9", "44:25.9", "44:25.9", "44:26.0", "44:26.0", "44:26.0", "44:26.1", "44:26.1", "44:26.1", "44:26.2", "44:26.2", "44:26.2", "44:26.3", "44:26.3", "44:26.3", "44:26.4", "44:26.4", "44:26.4", "44:26.5", "44:26.5", "44:26.5", "44:26.6", "44:26.6", "44:26.6", "44:26.7", "44:26.7", "44:26.7", "44:26.8", "44:26.8", "44:26.8", "44:26.9", "44:26.9", "44:26.9", "44:27.0", "44:27.0", "44:27.0", "44:27.1", "44:27.1", "44:27.1", "44:27.2", "44:27.2", "44:27.2", "44:27.3", "44:27.3", "44:27.3", "44:27.4", "44:27.4", "44:27.4", "44:27.5", "44:27.5", "44:27.5", "44:27.6", "44:27.6", "44:27.6", "44:27.7", "44:27.7", "44:27.7", "44:27.8", "44:27.8", "44:27.8", "44:27.9", "44:27.9", "44:27.9", "44:28.0", "44:28.0", "44:28.0", "44:28.1", "44:28.1", "44:28.1", "44:28.2", "44:28.2", "44:28.2", "44:28.3", "44:28.3", "44:28.3", "44:28.4", "44:28.4", "44:28.4", "44:28.5", "44:28.5", "44:28.5", "44:28.6", "44:28.6", "44:28.6", "44:28.7", "44:28.7", "44:28.7", "44:28.8", "44:28.8", "44:28.8", "44:28.9", "44:28.9", "44:28.9", "44:29.0", "44:29.0", "44:29.0", "44:29.1", "44:29.1", "44:29.1", "44:29.2", "44:29.2", "44:29.2", "44:29.3", "44:29.3", "44:29.3", "44:29.4", "44:29.4", "44:29.4", "44:29.5", "44:29.5", "44:29.5", "44:29.6", "44:29.6", "44:29.6", "44:29.7", "44:29.7", "44:29.7", "44:29.8", "44:29.8", "44:29.8", "44:29.9", "44:29.9", "44:29.9", "44:30.0", "44:30.0", "44:30.0", "44:30.1", "44:30.1", "44:30.1", "44:30.2", "44:30.2", "44:30.2", "44:30.3", "44:30.3", "44:30.3", "44:30.4", "44:30.4", "44:30.4", "44:30.5", "44:30.5", "44:30.5", "44:30.6", "44:30.6", "44:30.6", "44:30.7", "44:30.7", "44:30.7", "44:30.8", "44:30.8", "44:30.8", "44:30.9", "44:30.9", "44:30.9", "44:31.0", "44:31.0", "44:31.0", "44:31.1", "44:31.1", "44:31.1", "44:31.2", "44:31.2", "44:31.2", "44:31.3", "44:31.3", "44:31.3", "44:31.4", "44:31.4", "44:31.4", "44:31.5", "44:31.5", "44:31.5", "44:31.6", "44:31.6", "44:31.6", "44:31.7", "44:31.7", "44:31.7", "44:31.8", "44:31.8", "44:31.8", "44:31.9", "44:31.9", "44:31.9", "44:32.0", "44:32.0", "44:32.0", "44:32.1", "44:32.1", "44:32.1", "44:32.2", "44:32.2", "44:32.2", "44:32.3", "44:32.3", "44:32.3", "44:32.4", "44:32.4", "44:32.4", "44:32.5", "44:32.5", "44:32.5", "44:32.6", "44:32.6", "44:32.6", "44:32.7", "44:32.7", "44:32.7", "44:32.8", "44:32.8", "44:32.8", "44:32.9", "44:32.9", "44:32.9", "44:33.0", "44:33.0", "44:33.0", "44:33.1", "44:33.1", "44:33.1", "44:33.2", "44:33.2", "44:33.2", "44:33.3", "44:33.3", "44:33.3", "44:33.4", "44:33.4", "44:33.4", "44:33.5", "44:33.5", "44:33.5", "44:33.6", "44:33.6", "44:33.6", "44:33.7", "44:33.7", "44:33.7", "44:33.8", "44:33.8", "44:33.8", "44:33.9", "44:33.9", "44:33.9", "44:34.0", "44:34.0", "44:34.0", "44:34.1", "44:34.1", "44:34.1", "44:34.2", "44:34.2", "44:34.2", "44:34.3", "44:34.3", "44:34.3", "44:34.4", "44:34.4", "44:34.4", "44:34.5", "44:34.5", "44:34.5", "44:34.6", "44:34.6", "44:34.6", "44:34.7", "44:34.7", "44:34.7", "44:34.8", "44:34.8", "44:34.8", "44:34.9", "44:34.9", "44:34.9", "44:35.0", "44:35.0", "44:35.0", "44:35.1", "44:35.1", "44:35.1", "44:35.2", "44:35.2", "44:35.2", "44:35.3", "44:35.3", "44:35.3", "44:35.4", "44:35.4", "44:35.4", "44:35.5", "44:35.5", "44:35.5", "44:35.6", "44:35.6", "44:35.6", "44:35.7", "44:35.7", "44:35.7", "44:35.8", "44:35.8", "44:35.8", "44:35.9", "44:35.9", "44:35.9", "44:36.0", "44:36.0", "44:36.0", "44:36.1", "44:36.1", "44:36.1", "44:36.2", "44:36.2", "44:36.2", "44:36.3", "44:36.3", "44:36.3", "44:36.4", "44:36.4", "44:36.4", "44:36.5", "44:36.5", "44:36.5", "44:36.6", "44:36.6", "44:36.6", "44:36.7", "44:36.7", "44:36.7", "44:36.8", "44:36.8", "44:36.8", "44:36.9", "44:36.9", "44:36.9", "44:37.0", "44:37.0", "44:37.0", "44:37.1", "44:37.1", "44:37.1", "44:37.2", "44:37.2", "44:37.2", "44:37.3", "44:37.3", "44:37.3", "44:37.4", "44:37.4", "44:37.4", "44:37.5", "44:37.5", "44:37.5", "44:37.6", "44:37.6", "44:37.6", "44:37.7", "44:37.7", "44:37.7", "44:37.8", "44:37.8", "44:37.8", "44:37.9", "44:37.9", "44:37.9", "44:38.0", "44:38.0", "44:38.0", "44:38.1", "44:38.1", "44:38.1", "44:38.2", "44:38.2", "44:38.2", "44:38.3", "44:38.3", "44:38.3", "44:38.4", "44:38.4", "44:38.4", "44:38.5", "44:38.5", "44:38.5", "44:38.6", "44:38.6", "44:38.6", "44:38.7", "44:38.7", "44:38.7", "44:38.8", "44:38.8", "44:38.8", "44:38.9", "44:38.9", "44:38.9", "44:39.0", "44:39.0", "44:39.0", "44:39.1", "44:39.1", "44:39.1", "44:39.2", "44:39.2", "44:39.2", "44:39.3", "44:39.3", "44:39.3", "44:39.4", "44:39.4", "44:39.4", "44:39.5", "44:39.5", "44:39.5", "44:39.6", "44:39.6", "44:39.6", "44:39.7", "44:39.7", "44:39.7", "44:39.8", "44:39.8", "44:39.8", "44:39.9", "44:39.9", "44:39.9", "44:40.0", "44:40.0", "44:40.0", "44:40.1", "44:40.1", "44:40.1", "44:40.2", "44:40.2", "44:40.2", "44:40.3", "44:40.3", "44:40.3", "44:40.4", "44:40.4", "44:40.4", "44:40.5", "44:40.5", "44:40.5", "44:40.6", "44:40.6", "44:40.6", "44:40.7", "44:40.7", "44:40.7", "44:40.8", "44:40.8", "44:40.8", "44:40.9", "44:40.9", "44:40.9", "44:41.0", "44:41.0", "44:41.0", "44:41.1", "44:41.1", "44:41.1", "44:41.2", "44:41.2", "44:41.2", "44:41.3", "44:41.3", "44:41.3", "44:41.4", "44:41.4", "44:41.4", "44:41.5", "44:41.5", "44:41.5", "44:41.6", "44:41.6", "44:41.6", "44:41.7", "44:41.7", "44:41.7", "44:41.8", "44:41.8", "44:41.8", "44:41.9", "44:41.9", "44:41.9", "44:42.0", "44:42.0", "44:42.0", "44:42.1", "44:42.1", "44:42.1", "44:42.2", "44:42.2", "44:42.2", "44:42.3", "44:42.3", "44:42.3", "44:42.4", "44:42.4", "44:42.4", "44:42.5", "44:42.5", "44:42.5", "44:42.6", "44:42.6", "44:42.6", "44:42.7", "44:42.7", "44:42.7", "44:42.8", "44:42.8", "44:42.8", "44:42.9", "44:42.9", "44:42.9", "44:43.0", "44:43.0", "44:43.0", "44:43.1", "44:43.1", "44:43.1", "44:43.2", "44:43.2", "44:43.2", "44:43.3", "44:43.3", "44:43.3", "44:43.4", "44:43.4", "44:43.4", "44:43.5", "44:43.5", "44:43.5", "44:43.6", "44:43.6", "44:43.6", "44:43.7", "44:43.7", "44:43.7", "44:43.8", "44:43.8", "44:43.8", "44:43.9", "44:43.9", "44:43.9", "44:44.0", "44:44.0", "44:44.0", "44:44.1", "44:44.1", "44:44.1", "44:44.2", "44:44.2", "44:44.2", "44:44.3", "44:44.3", "44:44.3", "44:44.4", "44:44.4", "44:44.4", "44:44.5", "44:44.5", "44:44.5", "44:44.6", "44:44.6", "44:44.6", "44:44.7", "44:44.7", "44:44.7", "44:44.8", "44:44.8", "44:44.8", "44:44.9", "44:44.9", "44:44.9", "44:45.0", "44:45.0", "44:45.0", "44:45.1", "44:45.1", "44:45.1", "44:45.2", "44:45.2", "44:45.2", "44:45.3", "44:45.3", "44:45.3", "44:45.4", "44:45.4", "44:45.4", "44:45.5", "44:45.5", "44:45.5", "44:45.6", "44:45.6", "44:45.6", "44:45.7", "44:45.7", "44:45.7", "44:45.8", "44:45.8", "44:45.8", "44:45.9", "44:45.9", "44:45.9", "44:46.0", "44:46.0", "44:46.0", "44:46.1", "44:46.1", "44:46.1", "44:46.2", "44:46.2", "44:46.2", "44:46.3", "44:46.3", "44:46.3", "44:46.4", "44:46.4", "44:46.4", "44:46.5", "44:46.5", "44:46.5", "44:46.6", "44:46.6", "44:46.6", "44:46.7", "44:46.7", "44:46.7", "44:46.8", "44:46.8", "44:46.8", "44:46.9", "44:46.9", "44:46.9", "44:47.0", "44:47.0", "44:47.0", "44:47.1", "44:47.1", "44:47.1", "44:47.2", "44:47.2", "44:47.2", "44:47.3", "44:47.3", "44:47.3", "44:47.4", "44:47.4", "44:47.4", "44:47.5", "44:47.5", "44:47.5", "44:47.6", "44:47.6", "44:47.6", "44:47.7", "44:47.7", "44:47.7", "44:47.8", "44:47.8", "44:47.8", "44:47.9", "44:47.9", "44:47.9", "44:48.0", "44:48.0", "44:48.0", "44:48.1", "44:48.1", "44:48.1", "44:48.2", "44:48.2", "44:48.2", "44:48.3", "44:48.3", "44:48.3", "44:48.4", "44:48.4", "44:48.4", "44:48.5", "44:48.5", "44:48.5", "44:48.6", "44:48.6", "44:48.6", "44:48.7", "44:48.7", "44:48.7", "44:48.8", "44:48.8", "44:48.8", "44:48.9", "44:48.9", "44:48.9", "44:49.0", "44:49.0", "44:49.0", "44:49.1", "44:49.1", "44:49.1", "44:49.2", "44:49.2", "44:49.2", "44:49.3", "44:49.3", "44:49.3", "44:49.4", "44:49.4", 
